vi "New Message.vi"(8 "error in (no error)":errorcluster, 10 "Method Qualified Name":string, 11 "Message Maker in":refnum<class "Message Maker.lvclass">) -> (0 "error out":errorcluster, 1 "AF Library FQN":string, 2 "References":T1, 3 "Message Maker out":refnum<class "Message Maker.lvclass">, 4 "Updating?":bool)   [LabVIEW 2023, in "Message Maker.lvclass"]
doc: "Sets up the method to be built. If this is a new message, it will copy over the template. If this is a message to be updated it resets the old message\n\nAuthor: Derek Trepanier\nCopyright: MGI 2015"
uses:
  Message Maker.lvclass
  Message Maker.lvclass/Message Maker.ctl
  Scripting Refs.ctl
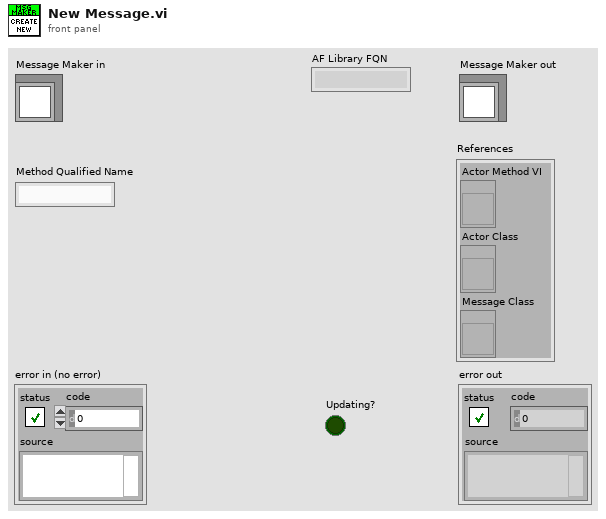
[diagram p1: front panel]
types:
  T1 = typedef "Message Maker.lvclass/Scripting Refs.ctl" = cluster{"Actor Method VI":refnum<vi>, "Actor Class":refnum<vi>, "Message Class":refnum<vi>}
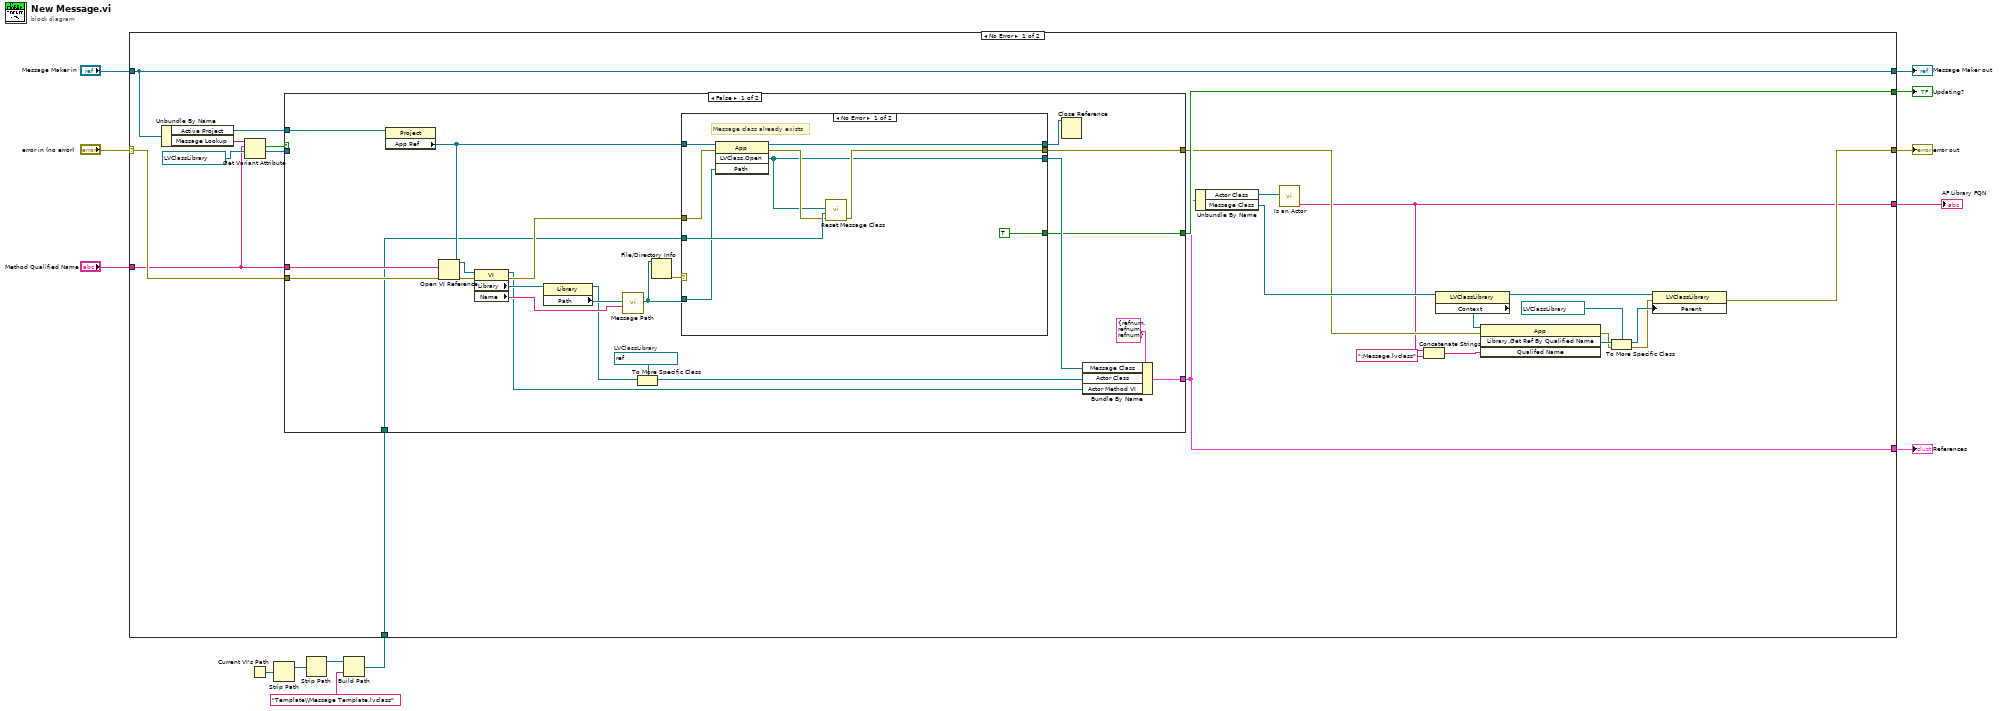
[diagram p0: block diagram]
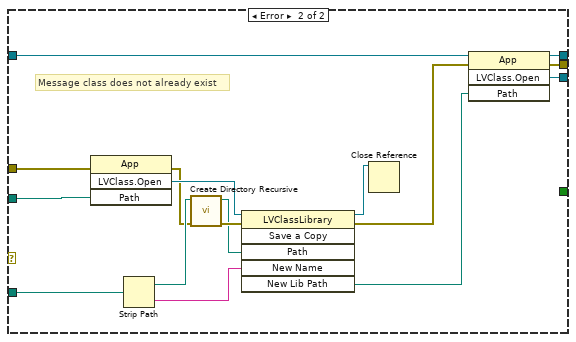
[diagram p2: hidden frame]
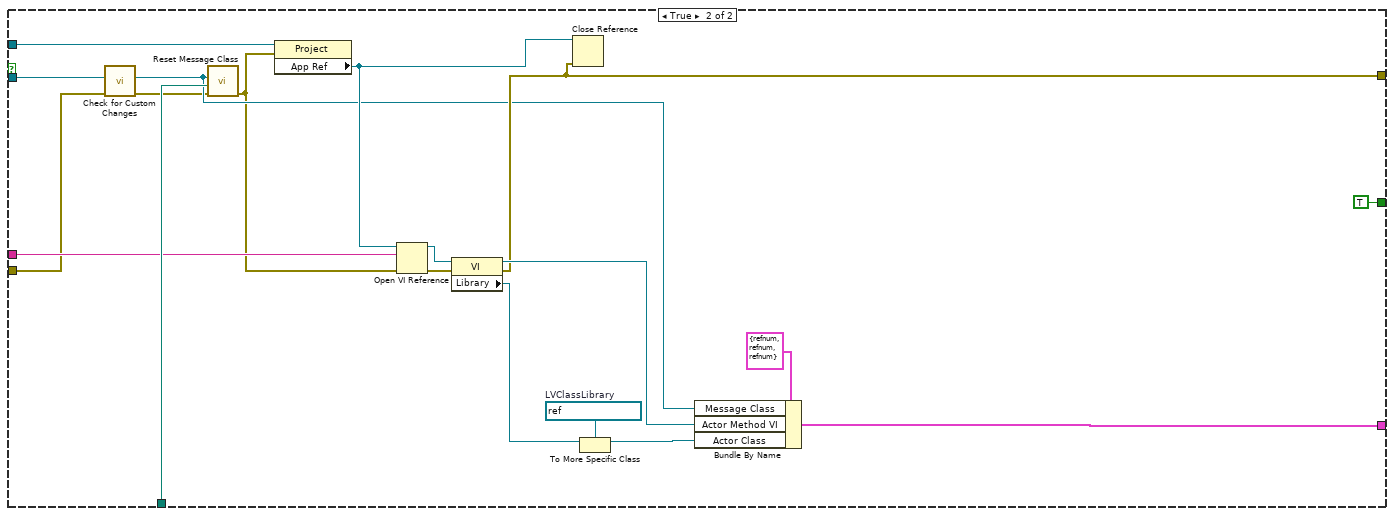
[diagram p3: hidden frame]
diagram:
  n1 = Current VI's Path() -> (path=w7:path)
  n2 = Strip Path(path=w7) -> (stripped path=w6:path)  [unwired: 1 out]
  n3 = Strip Path(path=w6) -> (stripped path=w5:path)  [unwired: 1 out]
  n4 = Build Path(base path=w5, name or relative path="Template\\Message Template.lvclass") -> (appended path=w3:path)
  n5 = case shown="No Error" "error in (no error)" {
    selector: "error in (no error)" -> [w36 w106]
    tunnel: [w25 w106] -> w12
    tunnel: [w38 w105] -> w10
    tunnel: "Message Maker in" -> [w38 w105]
    tunnel: "Method Qualified Name" -> [w33 _]
    tunnel: [w28 _] -> w8
    tunnel: w3 -> [w30 _]
    tunnel: [w29 _] -> w2
    tunnel: [w16 _] -> w1
    frame No Error {
      n6 = Unbundle By Name(w38) -> ("Active Project"=w37:refnum<vi>, "Message Lookup"=w35:variant)
      n7 = Get Variant Attribute(Variant=w35, name=w33, default value (empty Variant)=refnum<vi> refnum ("reference out")) -> (found=w32:bool, value=w31:refnum<vi>)  [unwired: 1 in, 2 out]
      n8 = case shown="False" w32 {
        tunnel: w37 -> [w59 w102]
        tunnel: [w52 w94] -> w28
        tunnel: w36 -> [w46 w89]
        tunnel: [w45 w92] -> w24
        tunnel: w33 -> [w43 w101]
        tunnel: w31 -> [_ w90]
        tunnel: w30 -> [w42 w104]
        tunnel: [w39 TRUE] -> w29
        frame False {
          w48 = refnum<vi> refnum  # LVClassLibrary
          n9 = property class="Project"(reference=w59) -> ("App Ref"=w54:refnum<vi>)  [unwired: 1 in, 2 out]
          n10 = Open VI Reference(application reference (local)=w54, vi path=w43, error in (no error)=w46) -> (vi reference=w60:refnum<vi>, error out=w61:errorcluster)  [unwired: 3 in]
          n11 = property class="VI"(reference=w60, error in=w61) -> (reference out=w51:refnum<vi>, error out=w55:errorcluster, "Library"=w58:refnum<vi>, "Name"=w56:string)
          n12 = property class="Library"(reference=w58) -> (reference out=w50:refnum<vi>, "Path"=w57:path)  [unwired: 1 in, 1 out]
          n13 = call "Message Path.vi"("Message Method"=w56, "Class Path"=w57) -> ("Message Class Path"=w41:path)  [unwired: 9 in]
          n14 = To More Specific Class(target class=w48, reference=w50) -> (specific class reference=w49:refnum<vi>)  [unwired: 1 in, 1 out]
          n15 = File/Directory Info(path=w41) -> (error out=w40:errorcluster)  [unwired: 1 in, 6 out]
          n16 = case shown="No Error" w40 {
            tunnel: w41 -> [w68 w80]
            tunnel: w55 -> [w65 w78]
            tunnel: w54 -> [w69 w77]
            tunnel: [w63 w74] -> w47
            tunnel: [w64 w73] -> w45
            tunnel: [w67 w72] -> w44
            tunnel: w42 -> [w70 w71]
            tunnel: [TRUE _] -> w39
            frame No Error {
              # "Message class already exists"
              n17 = invoke class="App" method="LVClass.Open"(reference=w69, error in=w65, "Path"=w68) -> (reference out=w67:refnum<vi>, error out=w66:errorcluster, "LVClass.Open"=w63:refnum<vi>)  [unwired: 1 in, 1 out]
              n18 = call "Reset Message Class.vi"("error in (no error)"=w66, "Template Path"=w70, "Message Class"=w63) -> ("error out"=w64:errorcluster)  [unwired: 8 in]
            }
            frame Error {
              # "Message class does not already exist"
              n19 = invoke class="App" method="LVClass.Open"(error in=w78, "Path"=w71) -> (error out=w79:errorcluster, "LVClass.Open"=w82:refnum<vi>)  [unwired: 2 in, 2 out]
              n20 = Strip Path(path=w80) -> (stripped path=w84:path, name=w81:string)
              n21 = call <vilib>:"Create Directory Recursive.vi"("error in (no error)"=w79, "directory"=w84) -> ("error out"=w86:errorcluster, "directory copy"=w85:path)  [unwired: 3 in, 1 out]
              n22 = invoke class="LVClassLibrary" method="Save a Copy"(reference=w82, error in=w86, "Path"=w85, "New Name"=w81) -> (reference out=w83:refnum<vi>, error out=w75:errorcluster, "New Lib Path"=w76:path)  [unwired: 2 in, 3 out]
              n23 = Close Reference(reference=w83) -> ()  [unwired: 1 in, 1 out]
              n24 = invoke class="App" method="LVClass.Open"(reference=w77, error in=w75, "Path"=w76) -> (reference out=w72:refnum<vi>, error out=w73:errorcluster, "LVClass.Open"=w74:refnum<vi>)  [unwired: 1 in, 1 out]
            }
          }
          n25 = Close Reference(reference=w44) -> ()  [unwired: 1 in, 1 out]
          n26 = Bundle By Name(cluster=T1 {"Actor Method VI"=refnum, "Actor Class"=refnum, "Message Class"=refnum} ("References"), "Message Class"=w47, "Actor Class"=w49, "Actor Method VI"=w51) -> (w52:T1)
        }
        frame True {
          w98 = refnum<vi> refnum  # LVClassLibrary
          n27 = call "Check for Custom Changes.vi"("error in (no error)"=w89, "Message Class"=w90) -> ("error out"=w88:errorcluster)  [unwired: 9 in]
          n28 = call "Reset Message Class.vi"("error in (no error)"=w88, "Template Path"=w104, "Message Class"=w90) -> ("error out"=w87:errorcluster)  [unwired: 8 in]
          n29 = property class="Project"(reference=w102, error in=w87) -> ("App Ref"=w93:refnum<vi>)  [unwired: 2 out]
          n30 = Open VI Reference(application reference (local)=w93, vi path=w101, error in (no error)=w87) -> (vi reference=w103:refnum<vi>, error out=w100:errorcluster)  [unwired: 3 in]
          n31 = property class="VI"(reference=w103, error in=w100) -> (reference out=w96:refnum<vi>, error out=w92:errorcluster, "Library"=w97:refnum<vi>)
          n32 = Close Reference(reference=w93, error in (no error)=w92) -> ()  [unwired: 1 out]
          n33 = To More Specific Class(target class=w98, reference=w97) -> (specific class reference=w95:refnum<vi>)  [unwired: 1 in, 1 out]
          n34 = Bundle By Name(cluster=T1 {"Actor Method VI"=refnum, "Actor Class"=refnum, "Message Class"=refnum} ("References"), "Message Class"=w90, "Actor Method VI"=w96, "Actor Class"=w95) -> (w94:T1)
        }
      }
      n35 = Unbundle By Name(w28) -> ("Actor Class"=w27:refnum<vi>, "Message Class"=w26:refnum<vi>)
      n36 = call "Is an Actor.vi"("Class in"=w27) -> ("AF Library FQN"=w16:string)  [unwired: 8 in, 2 out]
      n37 = Concatenate Strings(w16, ":Message.lvclass" ("string")) -> (w14:string)
      n38 = property class="LVClassLibrary"(reference=w26) -> (reference out=w23:refnum<vi>, "Context"=w22:refnum<vi>)  [unwired: 1 in, 1 out]
      n39 = invoke class="App" method="Library.Get Ref By Qualified Name"(reference=w22, error in=w24, "Qualifed Name"=w14) -> (error out=w18:errorcluster, "Library.Get Ref By Qualified Name"=w21:refnum<vi>)  [unwired: 1 in, 2 out]
      n40 = To More Specific Class(target class=refnum<vi> refnum ("Parent Class"), reference=w21, error in=w18) -> (specific class reference=w19:refnum<vi>, error out=w17:errorcluster)
      n41 = property class="LVClassLibrary"(reference=w23, error in=w17, "Parent"=w19) -> (error out=w25:errorcluster)  [unwired: 1 out]
    }
    frame Error {
    }
  }
  "error out" <- w12
  "Message Maker out" <- w10
  "References" <- w8
  "Updating?" <- w2
  "AF Library FQN" <- w1
